vi "IV_measure_DMM.vi"(8 "error in (no error)":errorcluster, 11 "Input parameters":T1={"Measurement type"=enum."Debug", "Sensor type"=enum."HPK_8in_271ch", "Identifier"="test.txt", "Open after execution?"=FALSE, "Plot after execution?"=FALSE, "Display channel"=0, "Voltage Delay (s)"=0.5, "Switch Delay (s)"=0.01, "VISA resource name source"="", "VISA resource name DMM"="", "VISA resource name LCR"="", "Compliance  Level (A)"=10.0, "Voltage Limit (V)"=1000.0, "Data storage location"="", "Scan voltages"="", "Use source as DMM?"=FALSE, "LCR signal frequenzy (Hz)"=10.0, "DMM device"=enum."Keithley2001", "Sampling number"=1, "Use env. sensors on"=enum."Sensirion sht1x/7x", "Switchboard Handle"=0, "Use Switchboard"=FALSE, "LCR signal voltage (V)"=10000.0, "Repeat"=1, "Scan voltages IV"="", "Scan voltages CV"="", "Hex pad numbers?"=FALSE, "Set measurement type"=enum."Debug", "Custom pad scan"="", "IV voltage Delay (s)"=0.5, "CV voltage Delay (s)"=0.5, "Needle measurement?"=FALSE, "Comments"="test.txt", "LCR signal frequenzy (kHz)"=10.0, "Compliance  Level (uA)"=10.0, "Open Correction Array"=array2304x3[6912 elements], "Current set voltage"=0.0, "Last set voltage"=0.0, "Current channel"=0, "Last OpenCorrection index"=-1, "Total curr/vltg every x steps"=10, "Current channel iteration"=0, "No CV corrections"=FALSE, "Mapfile"="", "Corrfile"="", "IV voltage file"=path "", "CV voltage file"=path "", "IV Switch Delay (s)"=0.01, "CV Switch Delay (s)"=0.01, "Invert polarity"=FALSE, "Set debug dirs"=FALSE, "Is n on p"=FALSE, "Source interlock?"=TRUE, "Voltage file used?"=FALSE, "Pad mask"="", "Mask pad above (uA)"=1.0, "LCR device"=enum."LCR_E4980", "Source device"=enum."Source_2410", "HexPlot binary path"="", "PadReductionFactor"=1.0, "Temperature degC"="", "Fluence [neq]"="", "Annealing [min]"=""} {"CV Switch Delay (s)" format="%#_13g"; "IV Switch Delay (s)" format="%#_13g"; "Last set voltage" format="%#_13g"; "Current set voltage" format="%#_13g"; "CV voltage Delay (s)" format="%#_13g"; "IV voltage Delay (s)" format="%#_13g"; "Voltage Limit (V)" format="%#_13g"; "Voltage Delay (s)" format="%#_13g"; "Switch Delay (s)" format="%#_13g"}) -> (0 "error out":errorcluster, 1 "Error":dbl, 2 "Result":dbl, 3 "Input parameters out":T1={"Measurement type"=enum."Debug", "Sensor type"=enum."HPK_8in_271ch", "Identifier"="test.txt", "Open after execution?"=FALSE, "Plot after execution?"=FALSE, "Display channel"=0, "Voltage Delay (s)"=0.5, "Switch Delay (s)"=0.01, "VISA resource name source"="", "VISA resource name DMM"="", "VISA resource name LCR"="", "Compliance  Level (A)"=10.0, "Voltage Limit (V)"=1000.0, "Data storage location"="", "Scan voltages"="", "Use source as DMM?"=FALSE, "LCR signal frequenzy (Hz)"=10.0, "DMM device"=enum."Keithley2001", "Sampling number"=1, "Use env. sensors on"=enum."Sensirion sht1x/7x", "Switchboard Handle"=0, "Use Switchboard"=FALSE, "LCR signal voltage (V)"=10000.0, "Repeat"=1, "Scan voltages IV"="", "Scan voltages CV"="", "Hex pad numbers?"=FALSE, "Set measurement type"=enum."Debug", "Custom pad scan"="", "IV voltage Delay (s)"=0.5, "CV voltage Delay (s)"=0.5, "Needle measurement?"=FALSE, "Comments"="test.txt", "LCR signal frequenzy (kHz)"=10.0, "Compliance  Level (uA)"=10.0, "Open Correction Array"=array2304x3[6912 elements], "Current set voltage"=0.0, "Last set voltage"=0.0, "Current channel"=0, "Last OpenCorrection index"=-1, "Total curr/vltg every x steps"=10, "Current channel iteration"=0, "No CV corrections"=FALSE, "Mapfile"="", "Corrfile"="", "IV voltage file"=path "", "CV voltage file"=path "", "IV Switch Delay (s)"=0.01, "CV Switch Delay (s)"=0.01, "Invert polarity"=FALSE, "Set debug dirs"=FALSE, "Is n on p"=FALSE, "Source interlock?"=TRUE, "Voltage file used?"=FALSE, "Pad mask"="", "Mask pad above (uA)"=1.0, "LCR device"=enum."LCR_E4980", "Source device"=enum."Source_2410", "HexPlot binary path"="", "PadReductionFactor"=1.0, "Temperature degC"="", "Fluence [neq]"="", "Annealing [min]"=""} {"CV Switch Delay (s)" format="%#_13g"; "IV Switch Delay (s)" format="%#_13g"; "Last set voltage" format="%#_13g"; "Current set voltage" format="%#_13g"; "CV voltage Delay (s)" format="%#_13g"; "IV voltage Delay (s)" format="%#_13g"; "Voltage Limit (V)" format="%#_13g"; "Voltage Delay (s)" format="%#_13g"; "Switch Delay (s)" format="%#_13g"})   [LabVIEW 2020]
doc: "Measure current from DMM."
uses:
  input_params.ctl
  <instrlib>/Keithley 2450/Keithley 2450.lvlib
  <instrlib>/Keithley 24XX/Keithley 24XX.lvlib
  <instrlib>/Keithley 6517/Keithley 6517.lvlib
  <instrlib>/Keithley 648X Series/Keithley 648X Series.lvlib
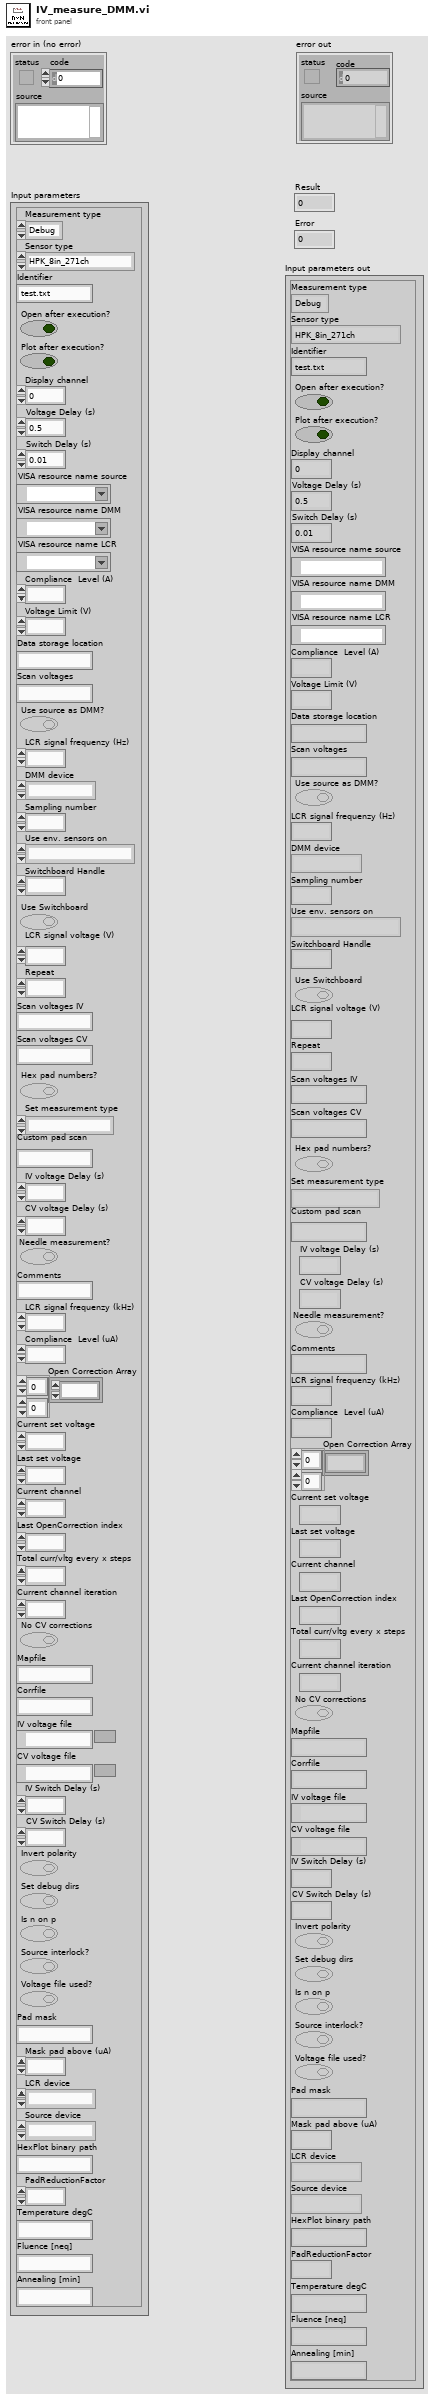
[diagram p1: front panel]
types:
  T1 = typedef "input_params.ctl" = cluster{"Measurement type":enum16{"IV", "CV", "Debug", "Test_contact"}, "Sensor type":enum16{"HPK_6in_135ch", "HPK_8in_271ch", "IFX_8in_256ch", "Diode", "HPK_6in_239ch", "Full_Matrix", "HPK_8in_271ch_full", "LumiCal", "HPK_8in_444ch", "HPK_8in_198ch_2019", "HPK_8in_MGW_LD_full", "HPK_8in_MGW_LD_a_type_top", "HPK_8in_MGW_LD_a_type_bottom", "HPK_8in_MGW_LD_b_type_left", "HPK_8in_MGW_LD_b_type_right", "HPK_8in_MGW_LD_c_type_left", "HPK_8in_MGW_LD_c_type_right", "HPK_8in_MGW_HD_full", "HPK_8in_MGW_HD_a_type_top", "HPK_8in_MGW_HD_a_type_bottom", "HPK_8in_MGW_HD_b_type_left", "HPK_8in_MGW_HD_b_type_right", "HPK_8in_MGW_HD_c_type_left", "HPK_8in_MGW_HD_c_type_right", "CALICE_6in_256ch"}, "Identifier":string, "Open after execution?":bool, "Plot after execution?":bool, "Display channel":i32, "Voltage Delay (s)":dbl, "Switch Delay (s)":dbl, "VISA resource name source":refnum<visa-resource-name>, "VISA resource name DMM":refnum<visa-resource-name>, "VISA resource name LCR":refnum<visa-resource-name>, "Compliance  Level (A)":dbl, "Voltage Limit (V)":dbl, "Data storage location":string, "Scan voltages":string, "Use source as DMM?":bool, "LCR signal frequenzy (Hz)":dbl, "DMM device":enum16{"Keithley2001", "Keithley2450", "Keithley2410", "Keithley6485", "Keithley6487", "Keithley6517"}, "Sampling number":i32, "Use env. sensors on":enum16{"Sensirion sht1x/7x", "Switch Matrix", "Probecard"}, "Switchboard Handle":u32, "Use Switchboard":bool, "LCR signal voltage (V)":dbl, "Repeat":i32, "Scan voltages IV":string, "Scan voltages CV":string, "Hex pad numbers?":bool, "Set measurement type":enum16{"IV", "CV", "Debug", "Test_contact", "IV+CV"}, "Custom pad scan":string, "IV voltage Delay (s)":dbl, "CV voltage Delay (s)":dbl, "Needle measurement?":bool, "Comments":string, "LCR signal frequenzy (kHz)":dbl, "Compliance  Level (uA)":dbl, "Open Correction Array":dbl[][], "Current set voltage":dbl, "Last set voltage":dbl, "Current channel":i32, "Last OpenCorrection index":i32, "Total curr/vltg every x steps":i32, "Current channel iteration":i32, "No CV corrections":bool, "Mapfile":string, "Corrfile":string, "IV voltage file":path, "CV voltage file":path, "IV Switch Delay (s)":dbl, "CV Switch Delay (s)":dbl, "Invert polarity":bool, "Set debug dirs":bool, "Is n on p":bool, "Source interlock?":bool, "Voltage file used?":bool, "Pad mask":string, "Mask pad above (uA)":dbl, "LCR device":enum16{"LCR_E4980", "AGILENT_4263X"}, "Source device":enum16{"Source_2410", "Source_6487", "Source_2470"}, "HexPlot binary path":string, "PadReductionFactor":dbl, "Temperature degC":string, "Fluence [neq]":string, "Annealing [min]":string}
  T2 = enum16{"Keithley2001", "Keithley2450", "Keithley2410", "Keithley6485", "Keithley6487", "Keithley6517"}
  T3 = cluster{"error":bool, "code":i32, "source":string}
  T4 = cluster{"Measurement":dbl, "Units":string, "Time Stamp and Date":string, "Reading #":dbl, "Channel #":dbl}
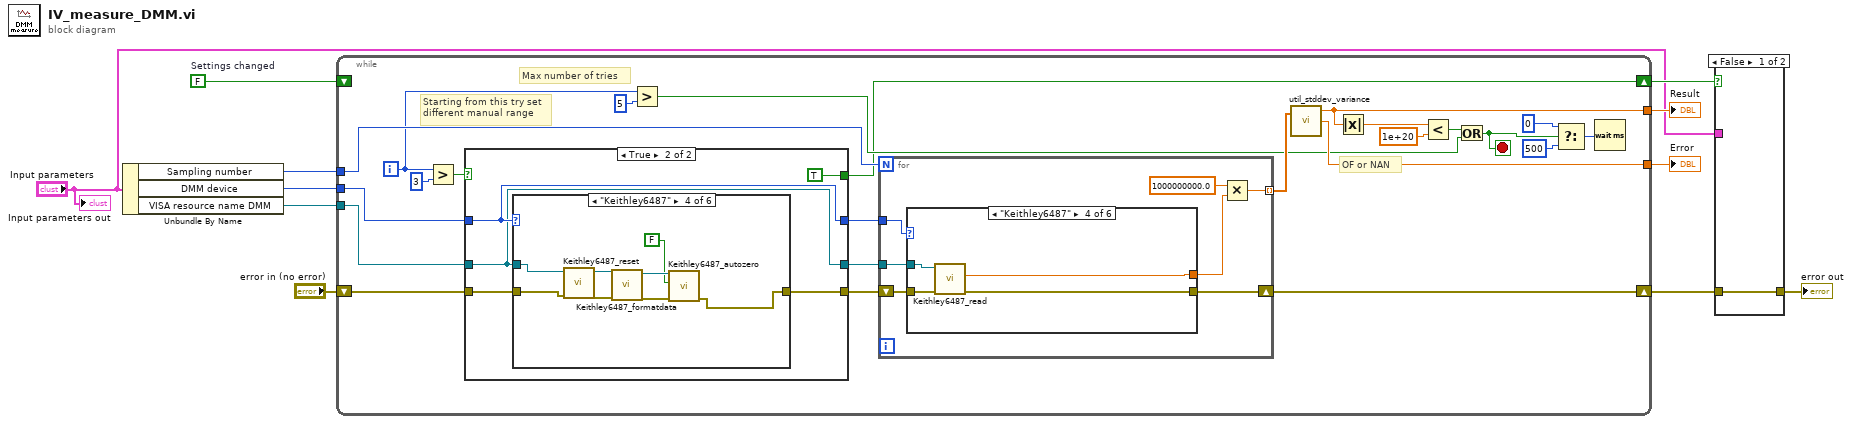
[diagram p0: block diagram]
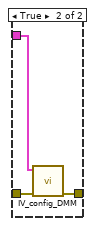
[diagram p2: hidden frame]
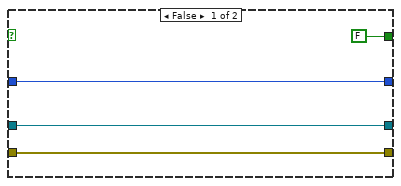
[diagram p3: hidden frame]
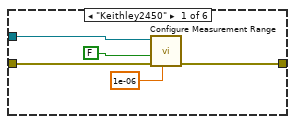
[diagram p4: hidden frame]
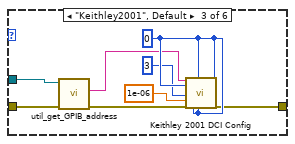
[diagram p6: hidden frame]
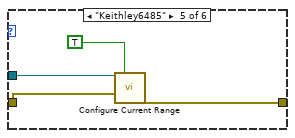
[diagram p7: hidden frame]
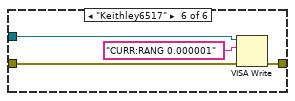
[diagram p8: hidden frame]
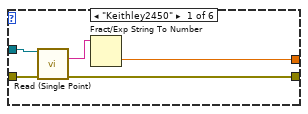
[diagram p9: hidden frame]
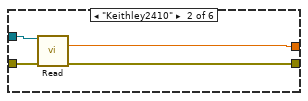
[diagram p10: hidden frame]
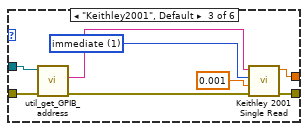
[diagram p11: hidden frame]
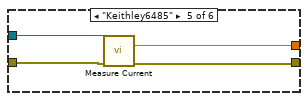
[diagram p12: hidden frame]
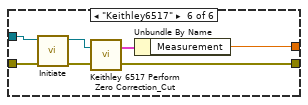
[diagram p13: hidden frame]
diagram:
  w5 = FALSE  # Settings changed
  n1 = Unbundle By Name("Input parameters") -> ("Sampling number"=w8:i32, "DMM device"=w11:T2, "VISA resource name DMM"=w10:refnum<visa-resource-name>)
  n2 = while {
    tunnel: w11 -> [w15]
    tunnel: w10 -> [w21]
    tunnel: w8 -> [w34]
    tunnel: [w32] -> w7
    tunnel: [w31] -> w6
    shift-right: [w35] -> w2
    shift-left: "error in (no error)" -> [w17]
    shift-right: [w12] -> w4
    shift-left: w5 -> [_]
    i -> [w20]
    stop <- w25 stop-if-true
    # "Starting from this try set\ndifferent manual range"
    # "OF or NAN"
    # "Max number of tries"
    n3 = Greater?(x=w20, y=3) -> (0:w18:bool)
    n4 = case shown="True" w18 {
      tunnel: w21 -> [w39 w42]
      tunnel: w17 -> [w38 w44]
      tunnel: [w38 w41] -> w16
      tunnel: w15 -> [w37 w43]
      tunnel: [w37 w43] -> w14
      tunnel: [w39 w42] -> w13
      tunnel: [FALSE TRUE] -> w12
      frame False {
      }
      frame True {
        n5 = case shown="\"Keithley6487\"" w43 {
          tunnel: w44 -> [w48 w50 w56 w63 w68 w74]
          tunnel: w42 -> [w49 _ w57 w66 w69 w73]
          tunnel: [w47 w50 w53 w59 w67 w72] -> w41
          frame "Keithley2450" {
            n6 = call <instrlib>:"Configure Measurement Range.vi"("Manual Range (1.0)"=1e-06, "error in (no error)"=w48, "Enable Auto Range (T:Enable)"=FALSE, "VISA resource name"=w49) -> ("error out"=w47:errorcluster)  [unwired: 6 in, 1 out]
          }
          frame "Keithley2410" {
          }
          frame "Keithley2001", Default {
            w58 = u16 0
            n7 = call "util_get_GPIB_address.vi"("error in (no error)"=w56, "VISA resource name"=w57) -> ("error out"=w54:errorcluster, "GPIB address"=w55:string)  [unwired: 7 in, 1 out]
            n8 = call <instrlib>:"Keithley 2001 DCI Config.vi"("GPIB address"=w55, "integration time (0:auto)"=w58, "range (auto:0)"=u16 3, "range value (amps)"=1e-06, "error in"=w54, "resolution (4.5 digits:3)"=w58, "reference (off:0)"=w58, "digital filter (off:0)"=w58, "advanced filter (off:0)"=w58) -> ("error out"=w53:T3)  [unwired: 10 in]
          }
          frame "Keithley6487" {
            n9 = call <instrlib>:"Keithley6487_reset.vi"("error in (no error)"=w63, "VISA resource name"=w66) -> ("error out"=w62:errorcluster, "VISA resource name out"=w65:refnum<visa-resource-name>)  [unwired: 8 in]
            n10 = call <instrlib>:"Keithley6487_formatdata.vi"("error in (no error)"=w62, "VISA resource name"=w65) -> ("error out"=w61:errorcluster, "VISA resource name out"=w64:refnum<visa-resource-name>)  [unwired: 8 in]
            n11 = call <instrlib>:"Keithley6487_autozero.vi"("error in (no error)"=w61, "Autozero"=FALSE, "VISA resource name"=w64) -> ("error out"=w59:errorcluster)  [unwired: 7 in, 1 out]
          }
          frame "Keithley6485" {
            n12 = call <instrlib>:"Configure Current Range.vi"("VISA resource name"=w69, "Autorange (T: Enable)"=TRUE, "error in (no error)"=w68) -> ("error out"=w67:errorcluster)  [unwired: 11 in, 1 out]
          }
          frame "Keithley6517" {
            n13 = VISA Write(VISA resource name=w73, write buffer="CURR:RANG 0.000001", error in (no error)=w74) -> (error out=w72:errorcluster)  [unwired: 2 out]
          }
        }
      }
    }
    n14 = Greater?(x=w20, y=5) -> (0:w28:bool)
    n15 = for {
      N: w34 -> [_]
      tunnel: w14 -> [w80]
      tunnel: w13 -> [w79]
      tunnel: [w75] -> w33 mode=indexing
      shift-right: [w81] -> w35
      shift-left: w16 -> [w78]
      n16 = case shown="\"Keithley6487\"" w80 {
        tunnel: w78 -> [w85 w90 w95 w100 w105 w110]
        tunnel: w79 -> [w84 w87 w92 w101 w106 w109]
        tunnel: [w83 w89 w98 w99 w104 w107] -> w81
        tunnel: [w82 w88 w96 w102 w103 w108] -> w76
        frame "Keithley2450" {
          n17 = call <instrlib>:"Read (Single Point).vi"("VISA resource name"=w84, "error in (no error)"=w85) -> ("Data out"=w86:string, "error out"=w83:errorcluster)  [unwired: 11 in, 1 out]
          n18 = Fract/Exp String To Number(string=w86) -> (number=w82:dbl)  [unwired: 3 in, 1 out]
        }
        frame "Keithley2410" {
          n19 = call-poly <instrlib>:"Read.vi"("VISA resource name"=w87, "error in (no error)"=w90) -> ("Current"=w88:sgl, "error out"=w89:errorcluster)  [unwired: 7 in, 5 out]
        }
        frame "Keithley2001", Default {
          w91 = u16 1 items=["hold", "immediate", "timer", "manual", "bus", "trigger link", "external"] ("source (imm:1)")
          n20 = call "util_get_GPIB_address.vi"("error in (no error)"=w95, "VISA resource name"=w92) -> ("error out"=w94:errorcluster, "GPIB address"=w93:string)  [unwired: 7 in, 1 out]
          n21 = call <instrlib>:"Keithley 2001 Single Read.vi"("GPIB address"=w93, "source (imm:1)"=w91, "timer value (secs)"=0.001, "error in"=w94) -> ("measurement"=w96:dbl, "error out"=w98:T3)  [unwired: 4 out]
        }
        frame "Keithley6487" {
          n22 = call <instrlib>:"Keithley6487_read.vi"("error in (no error)"=w100, "VISA resource name"=w101) -> ("error out"=w99:errorcluster, "output"=w102:dbl)  [unwired: 7 in, 1 out]
        }
        frame "Keithley6485" {
          n23 = call <instrlib>:"Measure Current.vi"("VISA resource name"=w106, "error in (no error)"=w105) -> ("Measurement"=w103:dbl, "error out"=w104:errorcluster)  [unwired: 11 in, 1 out]
        }
        frame "Keithley6517" {
          n24 = call <instrlib>:"Initiate.vi"("error in (no error)"=w110, "VISA resource name"=w109) -> ("error out"=w112:errorcluster, "VISA resource name out"=w111:refnum<visa-resource-name>)  [unwired: 8 in]
          n25 = call <instrlib>:"Keithley 6517 Perform Zero Correction_Cut.vi"("Error In"=w112, "VISA resource name"=w111) -> ("Error Out"=w107:errorcluster, "Measurement"=w113:T4)
          n26 = Unbundle By Name(w113) -> ("Measurement"=w108:dbl)
        }
      }
      n27 = Multiply(x=1000000000.0, y=w76) -> (x*y=w75:dbl)
    }
    n28 = call "util_stddev_variance.vi"("X"=w33) -> ("mean"=w31:dbl, "standard deviation"=w32:dbl)  [unwired: 1 in, 1 out]
    n29 = Absolute Value(x=w31) -> (abs(x)=w30:dbl)
    n30 = Less?(x=w30, y=1e+20) -> (x < y?=w27:bool)
    n31 = Or(x=w27, y=w28) -> (x .or. y?=w25:bool)
    n32 = Select(t=0, s=w25, f=500) -> (s? t:f=w23:i32)
    n33 = Wait (ms)(milliseconds to wait=w23) -> ()  [unwired: 1 out]
  }
  "Result" <- w6
  "Error" <- w7
  n34 = case shown="False" w4 {
    tunnel: "Input parameters" -> [_ w117]
    tunnel: w2 -> [w114 w116]
    tunnel: [w114 w115] -> w1
    frame False {
    }
    frame True {
      n35 = call "IV_config_DMM.vi"("error in (no error)"=w116, "Input parameters"=w117) -> ("error out"=w115:errorcluster)  [unwired: 9 in]
    }
  }
  "error out" <- w1
  "Input parameters out" <- "Input parameters"
